vi "nível de gasolina(SubVI).vi"(11 "data in":string) -> (3 "Numeric":dbl)   [LabVIEW 2015]
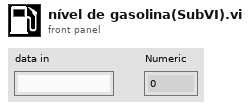
[diagram p1: front panel]
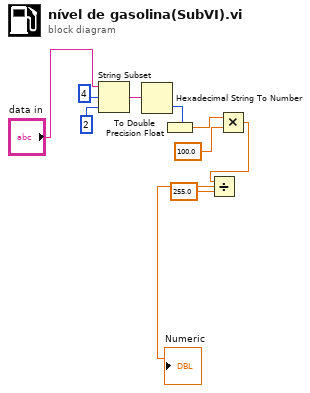
[diagram p0: block diagram]
diagram:
  n1 = String Subset(string="data in", offset (0)=4, length (rest)=2 ("length (rest)")) -> (substring=w4:string)
  n2 = Hexadecimal String To Number(string=w4) -> (number=w3:u32)  [unwired: 2 in, 1 out]
  n3 = To Double Precision Float(number=w3) -> (double precision float=w1:dbl)
  n4 = Multiply(x=w1, y=100.0) -> (x*y=w9:dbl)
  n5 = Divide(x=w9, y=255.0) -> (x/y=→"Numeric":dbl)
